vi "Read Channel Array.vi"(8 "error in":errorcluster, 10 "channels":refnum<class "Channel.lvclass">[](array[class]), 11 "digital output mode in":refnum<class "Digital Output Mode.lvclass">) -> (0 "error out":errorcluster, 2 "channel settings":T1[](array[typedef]), 3 "digital output mode out":refnum<class "Digital Output Mode.lvclass">)   [LabVIEW 2017, in "Scan Engine Scripting.lvlib" / "Digital Output Mode.lvclass"]
uses:
  Digital Output Mode.lvclass
  Channel Classes/Channel/Channel.lvclass
  Controls/digital channel settings.ctl
  Channel Classes/DO Channel/DO Channel.lvclass
  C:/Users/nitest/Documents/niveristand-scan-engine-ethercat-custom-device/Custom Device Source/Scripting/Modules/Channel Classes/Digital Channel/Digital Channel.lvclass
  Channel Classes/Digital Channel/Digital Channel.lvclass
  Scan Engine Scripting.lvlib
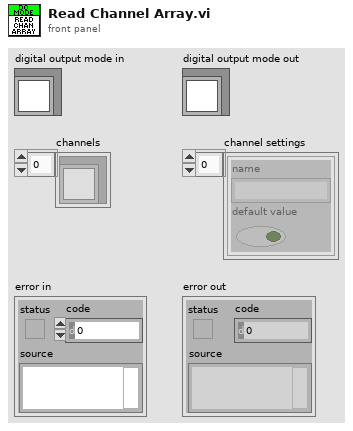
[diagram p1: front panel]
types:
  T1 = typedef "Scan Engine Scripting.lvlib/digital channel settings.ctl" = cluster{"name":string, "default value":bool}
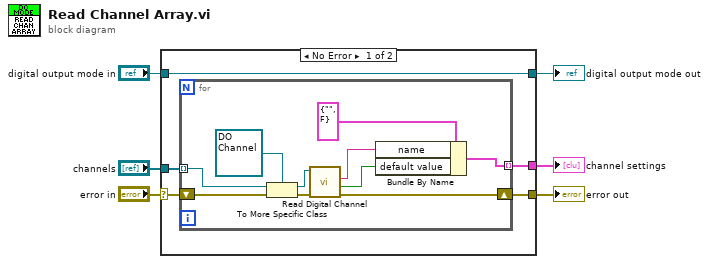
[diagram p0: block diagram]
diagram:
  n1 = case shown="No Error" "error in" {
    selector: "error in" -> [w9 w23]
    tunnel: [w8 w23] -> w5
    tunnel: [w11 w22] -> w3
    tunnel: "digital output mode in" -> [w11 w22]
    tunnel: "channels" -> [w10 _]
    tunnel: [w7 _] -> w1
    frame No Error {
      n2 = for {
        tunnel: w10 -> [w18] mode=indexing
        tunnel: [w20] -> w7 mode=indexing
        shift-right: [w14] -> w8
        shift-left: w9 -> [w19]
        n3 = To More Specific Class(target class=refnum<class "DO Channel.lvclass"> refnum ("Scan Engine Scripting.lvlib:DO Channel.lvclass"), reference=w18, error in=w19) -> (specific class reference=w15:refnum<class "DO Channel.lvclass">, error out=w16:errorcluster)
        n4 = call "Read Digital Channel.vi"("error in"=w16, "digital channel in"=w15) -> ("error out"=w14:errorcluster, "default value"=w13:bool, "name"=w12:string)  [unwired: 5 in, 2 out]
        n5 = Bundle By Name(cluster=T1 {"name"="", "default value"=FALSE} ("channel settings"), "name"=w12, "default value"=w13) -> (w20:T1)
      }
    }
    frame Error {
    }
  }
  "error out" <- w5
  "digital output mode out" <- w3
  "channel settings" <- w1
